vi "Capability Query.vi"(8 "error in (no error)":errorcluster, 11 "Refnum In":refnum<vi>) -> (0 "error out":errorcluster, 2 "Board Capability":map{i32, T1}(c390), 3 "Refnum Out":refnum<vi>)   [LabVIEW 2020, in "FirmataClient.lvlib"]
doc: "Retrieve the capability of all the pins of the currently connected board. This mainly includes the list of modes supported by each pin along with the resolution for the mode (i.e. a Pin supporting Analog Mode might have a resolution of 14bits)"
uses:
  FirmataClient.lvlib
  Controls/FirmataPinCapabilitiesAndAnalogMapping.ctl
  Controls/FirmataPinCapability.ctl
  Controls/FirmataPinModes.ctl
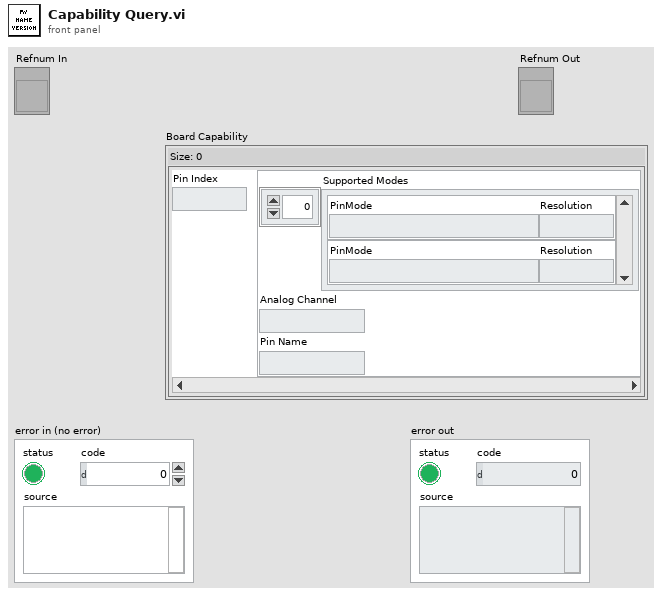
[diagram p1: front panel]
types:
  T1 = typedef "FirmataClient.lvlib/FirmataPinCapabilitiesAndAnalogMapping.ctl" = cluster{"Supported Modes":T2[], "Analog Channel":u8, "Pin Name":string}
  T2 = typedef "FirmataClient.lvlib/FirmataPinCapability.ctl" = cluster{"PinMode":T3, "Resolution":u8}
  T3 = typedef "FirmataClient.lvlib/FirmataPinModes.ctl" = enum16{"DigitalInput", "DigitalOutput", "AnalogInput", "PWM", "Servo", "Shift", "I2C", "OneWire", "Stepper", "Encoder", "Serial", "InputPullup", "Extended.SPI", "Extended.Sonar", "Extended.Tone", "Extended.DHT"}
  T4 = typedef "FirmataClient.lvlib/FirmataProtocolConstants.ctl" = u16
  T5 = typedef "FirmataClient.lvlib/Parameters.ctl" = cluster{"Transport Parameters":T6, "Board Capabilities":map{i32, T1}}
  T6 = typedef "FirmataClient.lvlib/TransportParameters.ctl" = cluster{"Serial Communication":cluster{"Comport":refnum<visa-resource-name>, "No Response Timeout Ms":u32, "Response Complete Timeout Ms":u32, "Max Rx Length":u32, "Baud Rate":u32}, "Selected Transport":T7, "Initializer File Path":path, "Cleaner File Path":path, "Transporter File Path":path}
  T7 = typedef "FirmataClient.lvlib/SupportedTransports.ctl" = enum16{"Serial Communication Port"}
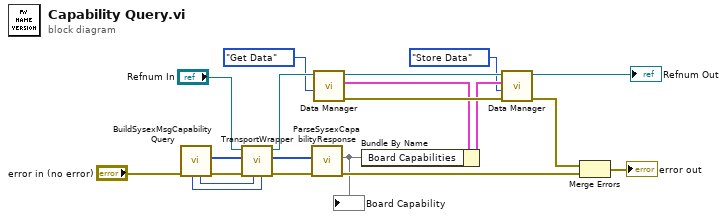
[diagram p0: block diagram]
diagram:
  n1 = call "BuildSysexMsgCapabilityQuery.vi"("error in"="error in (no error)") -> ("error out"=w20:errorcluster, "GetCapabilitiesMessage"=w15:u8[], "ReplyFirstByte"=w17:T4, "ReplyLength"=w16:i32)  [unwired: 7 in]
  n2 = call "TransportWrapper.vi"("ReplyLength"=w16, "ReplyFirstByte"=w17, "error in"=w20, "Message In"=w15, "Refnum In"="Refnum In") -> ("error out"=w14:errorcluster, "Message Out"=w13:u8[], "Refnum Out"=w12:refnum<vi>)  [unwired: 4 in]
  n3 = call "ParseSysexCapabilityResponse.vi"("error in"=w14, "Sysex Message"=w13) -> ("error out"=w7:errorcluster, "Map"=w4:map{i32, T1})  [unwired: 7 in, 1 out]
  "Board Capability" <- w4
  n4 = call "Data Manager.vi"("Mode"=enum16{"Store Data", "Get Data", "Cleanup"}."Get Data", "Refnum In"=w12) -> ("error out"=w9:errorcluster, "Data Out"=w5:T5, "Refnum Out"=w11:refnum<vi>)  [unwired: 7 in]
  n5 = Bundle By Name(cluster=w5, "Board Capabilities"=w4) -> (w3:T5)
  n6 = call "Data Manager.vi"("error in (no error)"=w9, "Mode"=enum16{"Store Data", "Get Data", "Cleanup"}."Store Data", "Data In"=w3, "Refnum In"=w11) -> ("error out"=w8:errorcluster, "Refnum Out"=→"Refnum Out":refnum<vi>)  [unwired: 5 in, 1 out]
  n7 = Merge Errors(w8, w7) -> (→"error out":errorcluster)
